vi "test sequencer parse sequence txt.vi"(8 "error in (no error)":errorcluster, 11 "sequence txt path":path) -> (0 "error out":errorcluster, 3 "steps":string[][](array[string]))   [LabVIEW 2019]
uses:
  <vilib>/Utility/file.llb/Read Delimited Spreadsheet (string).vi
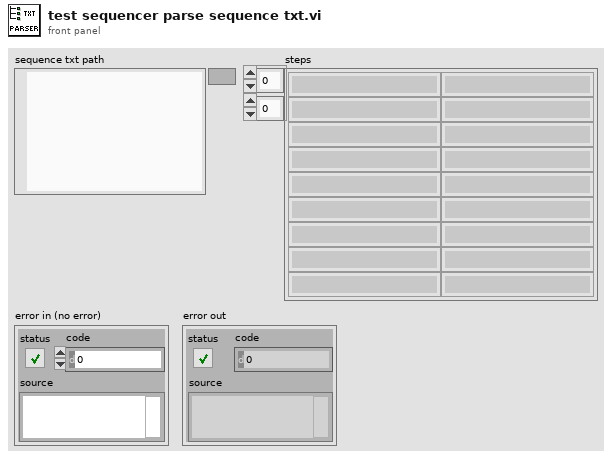
[diagram p1: front panel]
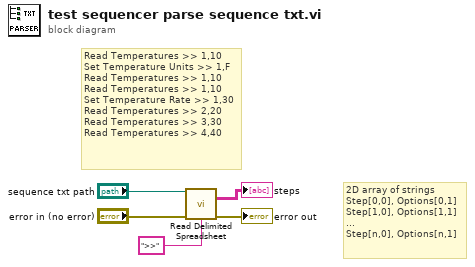
[diagram p0: block diagram]
diagram:
  # "2D array of strings\nStep[0,0], Options[0,1]\nStep[1,0], Options[1,1]\n...\nStep[n,0], Options[n,1]"
  # "Read Temperatures >> 1,10\nSet Temperature Units >> 1,F\nRead Temperatures >> 1,10\nRead Temperatures >> 1,10\nSet Temperature Rate >> 1,30\nRead Temperatures >> 2,20\nRead Temperatures >> 3,30\nRead Temperatures >> 4,40"
  n1 = call-poly <vilib>:"Read Delimited Spreadsheet.vi"("file path (dialog if empty)"="sequence txt path", "error in (no error)"="error in (no error)", "delimiter (\\t)"=">>" ("delimiter (\\t)")) -> ("all rows"=→"steps":string[][], "error out"=→"error out":errorcluster)  [unwired: 7 in, 4 out]
